vi "Remove LVProject.vi"(8 "error in (no error)":errorcluster, 10 "User Selections":string[](array[string]), 11 "BuildServer in":refnum<class "BuildServer.lvclass">) -> (0 "error out":errorcluster, 3 "BuildServer out":refnum<class "BuildServer.lvclass">)   [LabVIEW 2017, in "BuildServer.lvlib" / "BuildServer.lvclass"]
uses:
  BuildServer.lvclass
  C:/Program Files (x86)/National Instruments/LabVIEW 2017/vi.lib/ActorFramework/Actor/Actor.lvclass
  <vilib>/ActorFramework/Actor/Actor.lvclass/Actor.ctl
  <vilib>/ActorFramework/Message Enqueuer/Message Enqueuer.lvclass/Message Enqueuer.ctl
  BuildServer.lvclass/BuildServer.ctl
  <vilib>/ActorFramework/Message Enqueuer/Init from Existing Queue.vi
  <vilib>/ActorFramework/Message Enqueuer/Enqueue.vi
  BuildServer Messages/Update Tree Msg/Update Tree Msg.lvclass
  C:/Program Files (x86)/National Instruments/LabVIEW 2017/vi.lib/ActorFramework/Message/Message.lvclass
  <vilib>/ActorFramework/Message Priority Queue/Priority Enqueue.vi
  <vilib>/ActorFramework/Message Enqueuer/Message Enqueuer.lvclass
  <vilib>/BenjaminR/LookUp Table API/LUT.lvclass
  <vilib>/ActorFramework/Actor/Actor.lvclass
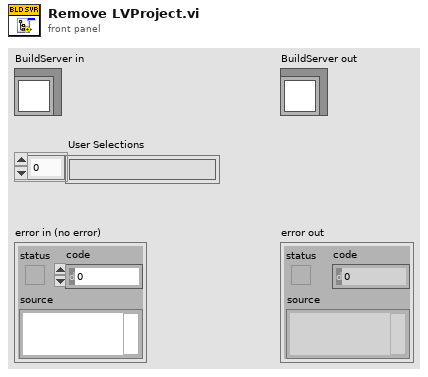
[diagram p1: front panel]
types:
  T1 = typedef "BuildServer.lvlib/BuildServer.lvclass/ProjectOrganization.ctl" = enum16{"Group by Project", "Group by Target", "Group by Type", "Group by Name"}
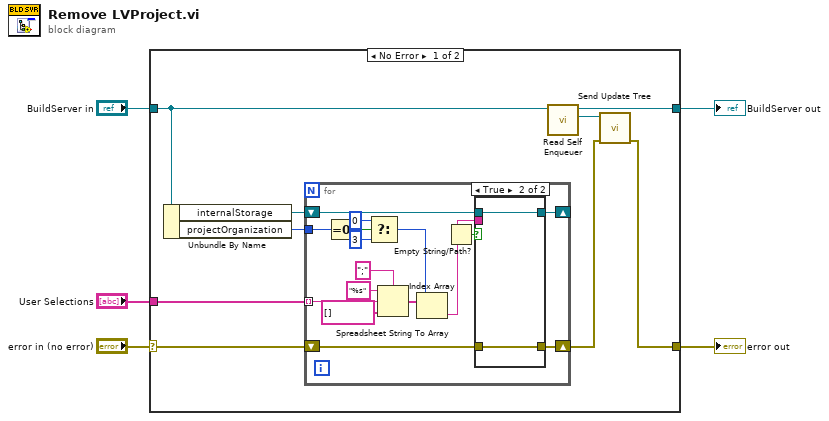
[diagram p0: block diagram]
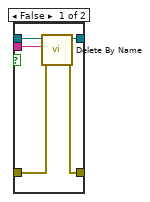
[diagram p2: hidden frame]
diagram:
  n1 = case shown="No Error" "error in (no error)" {
    selector: "error in (no error)" -> [w7 w38]
    tunnel: [w6 w38] -> w4
    tunnel: [w9 w37] -> w2
    tunnel: "BuildServer in" -> [w9 w37]
    tunnel: "User Selections" -> [w12 _]
    frame No Error {
      n2 = Unbundle By Name(w9) -> ("internalStorage"=w13:refnum<class "LUT.lvclass">, "projectOrganization"=w11:T1)
      n3 = for {
        shift-right: [w28] -> _
        shift-left: w13 -> [w29]
        tunnel: w12 -> [w27] mode=indexing
        tunnel: w11 -> [w21]
        shift-right: [w17] -> w8
        shift-left: w7 -> [w16]
        n4 = Equal To 0?(x=w21) -> (x = 0?=w22:bool)
        n5 = Select(t=0 ("index"), s=w22, f=3 ("index")) -> (s? t:f=w18:i32)
        n6 = Spreadsheet String To Array(delimiter (Tab)=";", format string="%s", spreadsheet string=w27, array type (2D Dbl)=string[] []) -> (array=w24:string[])
        n7 = Index Array(array=w24, index=w18) -> (element=w15:string)
        n8 = Empty String/Path?(string/path=w15) -> (empty?=w14:bool)
        n9 = case shown="True" w14 {
          tunnel: w29 -> [w34 w36]
          tunnel: [w33 w36] -> w28
          tunnel: [w32 w35] -> w17
          tunnel: w16 -> [w31 w35]
          tunnel: w15 -> [w30 _]
          frame False {
            n10 = call <vilib>:"Delete By Name.vi"("error in (no error)"=w31, "Name"=w30, "LUT in"=w34) -> ("error out"=w32:errorcluster, "LUT out"=w33:refnum<class "LUT.lvclass">)  [unwired: 6 in, 1 out]
          }
          frame True {
          }
        }
      }
      n11 = call <vilib>:"Read Self Enqueuer.vi"("Actor"=w9) -> ("Self Enqueuer"=w10:refnum<class "Message Enqueuer.lvclass">)  [unwired: 10 in]
      n12 = call "Send Update Tree.vi"("error in (no error)"=w8, "Message Enqueuer in"=w10) -> ("error out"=w6:errorcluster)  [unwired: 8 in, 1 out]
    }
    frame Error {
    }
  }
  "error out" <- w4
  "BuildServer out" <- w2
